vi "clear_buffers.vi"(8 "error in (no error)":errorcluster, 11 "FPGAWrapperRK120511Fiber_Spiral in":refnum<class "FPGAWrapperRK110512Fiber_Spiral.lvclass">) -> (0 "error out":errorcluster, 3 "FPGAWrapperRK120511Fiber_Spiral out":refnum<class "FPGAWrapperRK110512Fiber_Spiral.lvclass">)   [LabVIEW 2010, in "FPGAWrapperRK110512Fiber_Spiral.lvclass"]
uses:
  FPGAWrapperRK110512Fiber_Spiral.lvclass
  <vilib>/rvi/interface/nirviMethod/nirviMethod.xnode
  FPGA_VI_Reference.ctl
  <vilib>/Utility/error.llb/Error Cluster From Error Code.vi
  NiFpgaLv.dll
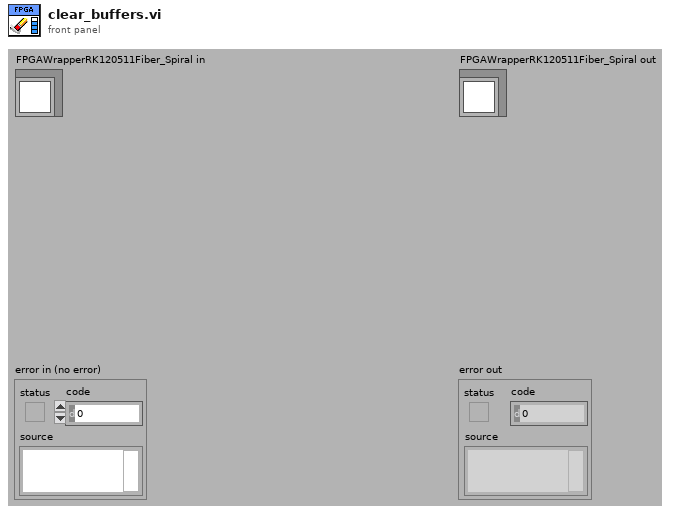
[diagram p1: front panel]
types:
  T1 = typedef "FPGAWrapperRK110512Fiber_Spiral.lvclass/FPGA_VI_Reference.ctl" = refnum<k20>
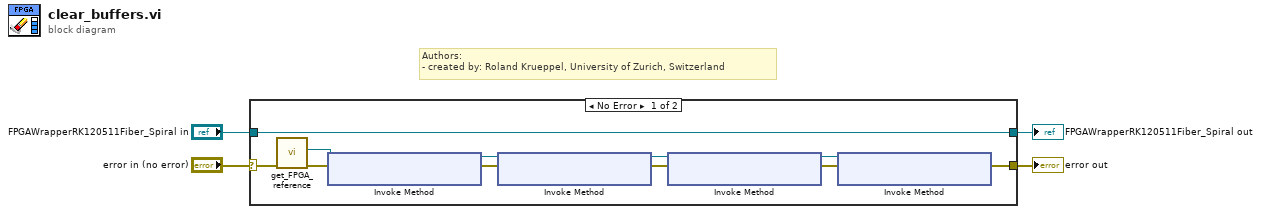
[diagram p0: block diagram]
diagram:
  # "Authors: \n- created by: Roland Krueppel, University of Zurich, Switzerland"
  n1 = case shown="No Error" "error in (no error)" {
    selector: "error in (no error)" -> [w15 w105]
    tunnel: [w6 w105] -> w3
    tunnel: "FPGAWrapperRK120511Fiber_Spiral in" -> [w5 w104]
    tunnel: [w5 w104] -> w1
    frame No Error {
      n2 = call "get_FPGA_reference.vi"("error in (no error)"=w15) -> ("error out"=w14:errorcluster, "FPGA VI Reference"=w13:T1)  [unwired: 8 in, 1 out]
      n3 = xnode "Invoke Method"("FPGA VI Reference In"=w13, "error in"=w14) -> ("FPGA VI Reference Out"=w11:T1, "error out"=w12:errorcluster)
      n4 = xnode "Invoke Method"("FPGA VI Reference In"=w11, "error in"=w12) -> ("FPGA VI Reference Out"=w9:T1, "error out"=w10:errorcluster)
      n5 = xnode "Invoke Method"("FPGA VI Reference In"=w9, "error in"=w10) -> ("FPGA VI Reference Out"=w7:T1, "error out"=w8:errorcluster)
      n6 = xnode "Invoke Method"("FPGA VI Reference In"=w7, "error in"=w8) -> ("error out"=w6:errorcluster)  [unwired: 1 out]
    }
    frame Error {
    }
  }
  "error out" <- w3
  "FPGAWrapperRK120511Fiber_Spiral out" <- w1
